vi "apply key value pairs.vi"(8 "error in":errorcluster, 9 "values":string[](array[string]), 10 "keys":string[](array[string]), 11 "fixed channel runtime in":refnum<class "State Machine runtime.lvclass">) -> (0 "error out":errorcluster, 3 "fixed channel runtime out":refnum<class "State Machine runtime.lvclass">)   [LabVIEW 2021, in "State Machine runtime.lvclass"]
uses:
  State Machine runtime.lvclass
  State Machine runtime.lvclass/State Machine runtime.ctl
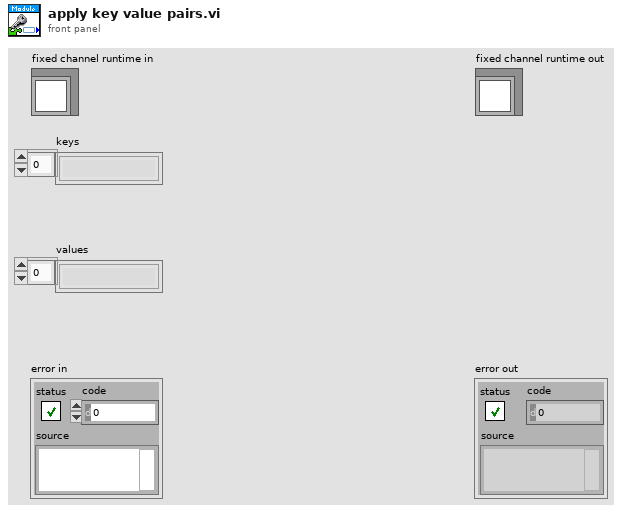
[diagram p1: front panel]
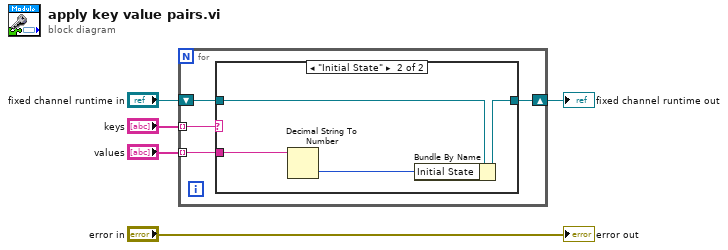
[diagram p0: block diagram]
diagram:
  n1 = for {
    tunnel: "keys" -> [w9] mode=indexing
    shift-right: [w8] -> w3
    shift-left: "fixed channel runtime in" -> [w7]
    tunnel: "values" -> [w6] mode=indexing
    n2 = case shown="\"Initial State\"" w9 {
      tunnel: [w10 w13] -> w8
      tunnel: w7 -> [w10 w14]
      tunnel: w6 -> [_ w12]
      frame Default {
      }
      frame "Initial State" {
        n3 = Decimal String To Number(string=w12) -> (number=w11:i32)  [unwired: 2 in, 1 out]
        n4 = Bundle By Name(cluster=w14, "Initial State"=w11) -> (w13:refnum<class "State Machine runtime.lvclass">)
      }
    }
  }
  "fixed channel runtime out" <- w3
  "error out" <- "error in"
